vi "norm.vi"(1 "amplitude matrix":cdb[][](array[numeric]) format="%.2f") -> (0 "norm":dbl format="%.2f")   [LabVIEW 2024]
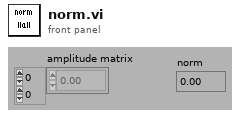
[diagram p1: front panel]
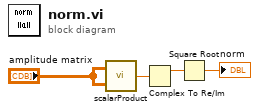
[diagram p0: block diagram]
diagram:
  n1 = call "scalarProduct.vi"("amplitude matrix 2"="amplitude matrix", "amplitude matrix 1"="amplitude matrix") -> ("scalar product"=w3:cdb)
  n2 = Complex To Re/Im(x + iy=w3) -> (x=w1:dbl)  [unwired: 1 out]
  n3 = Square Root(x=w1) -> (sqrt(x)=→"norm":dbl)
